vi "get_OEMCP.vi"(8 "error in (no error)":errorcluster) -> (0 "error out":errorcluster, 3 "OEMCodePage":i32)   [LabVIEW 2015, in "dotnet_system_exec.lvclass"]
doc: "Reads the OEMCP value into registry key HKLM\\SYSTEM\\CurrentControlSet\\Control\\Nls\\CodePage and returns the code page value as numeric."
uses:
  dotnet_system_exec.lvclass
  <vilib>/registry/registry.llb/Registry SAM.ctl
  <vilib>/registry/registry.llb/Read Registry Value Simple STR.vi
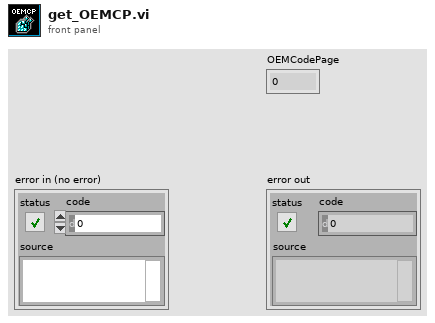
[diagram p1: front panel]
types:
  T1 = typedef "Registry SAM.ctl" = enum32{"KEY_QUERY_VALUE", "KEY_SET_VALUE", "KEY_CREATE_SUB_KEY", "KEY_ENUMERATE_SUB_KEYS", "KEY_NOTIFY", "KEY_CREATE_LINK", "KEY_READ", "KEY_WRITE", "KEY_ALL_ACCESS", "KEY_READ | KEY_WRITE"}
  T2 = typedef "Registry refnum.ctl" = refnum<k1>
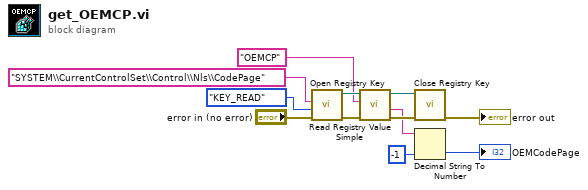
[diagram p0: block diagram]
diagram:
  n1 = call <vilib>:"Open Registry Key.vi"("error in (no error)"="error in (no error)", "security access mask (KEY_READ | KEY_WRITE)"=Registry_SAM."KEY_READ", "subkey"="SYSTEM\\CurrentControlSet\\Control\\Nls\\CodePage") -> ("error out"=w7:errorcluster, "refnum out"=w12:T2)  [unwired: 7 in]
  n2 = call-poly <vilib>:"Read Registry Value Simple.vi"("error in (no error)"=w7, "value"="OEMCP", "refnum"=w12) -> ("error out"=w6:errorcluster, "String/Binary data"=w4:string, "refnum out"=w9:T2)  [unwired: 3 in, 1 out]
  n3 = call <vilib>:"Close Registry Key.vi"("error in (no error)"=w6, "refnum"=w9) -> ("error out"=→"error out":errorcluster)  [unwired: 5 in]
  n4 = Decimal String To Number(string=w4, default (0L)=-1 ("default (0 I32)")) -> (number=→"OEMCodePage":i32)  [unwired: 1 in, 1 out]
